vi "Teleop.vi"(10 "Match Info":T1={"Autonomous Elapsed Seconds"=0.0, "TeleOp Elapsed Seconds"=0.0, "Disabled Elapsed Seconds"=0.0, "Visited Autonomous"=FALSE, "Visited TeleOp"=FALSE, "Visited Disabled"=FALSE, "Autonomous Settings"={"Autonomous Style"=enum."Independent", "VI Refnum"=refnum}}, 11 "Call Context":T2) -> ()   [LabVIEW 2014]
doc: "This VI is called for each TeleOp packet received from the DS where the robot is not disabled. It is often used to read from the joysticks and update I/O or to update setpoints for timed control loops. It should complete and return within 20 milliseconds or it may miss DS packets."
uses:
  <vilib>/Rock Robotics/WPI/DriverStation/WPI_DriverStationDerivedRobotMode.ctl
  <vilib>/Rock Robotics/WPI/DriverStation/WPI_DriverStationMatch Info.ctl
  <vilib>/Rock Robotics/Network Tables/SD Read Boolean.vi
  <vilib>/Rock Robotics/Network Tables/SD Read Number.vi
  <vilib>/Rock Robotics/Network Tables/SD Write Numeric Array.vi
panel:
  out "Sample Slider 0":dbl(slide) scale=0.0..5.0
  out "Sample Boolean 1":bool
  out "Sample Boolean 0":bool
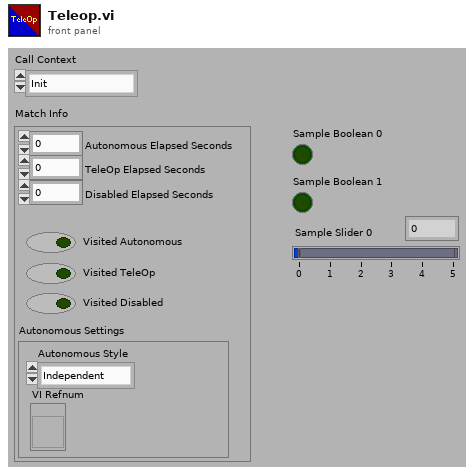
[diagram p1: front panel]
types:
  T1 = typedef "WPI_DriverStationMatch Info.ctl" = cluster{"Autonomous Elapsed Seconds":dbl, "TeleOp Elapsed Seconds":dbl, "Disabled Elapsed Seconds":dbl, "Visited Autonomous":bool, "Visited TeleOp":bool, "Visited Disabled":bool, "Autonomous Settings":cluster{"Autonomous Style":enum16{"Iterative", "Independent"}, "VI Refnum":refnum<vi>}}
  T2 = typedef "WPI_DriverStationDerivedRobotMode.ctl" = enum16{"Init", "Execute", "Stop"}
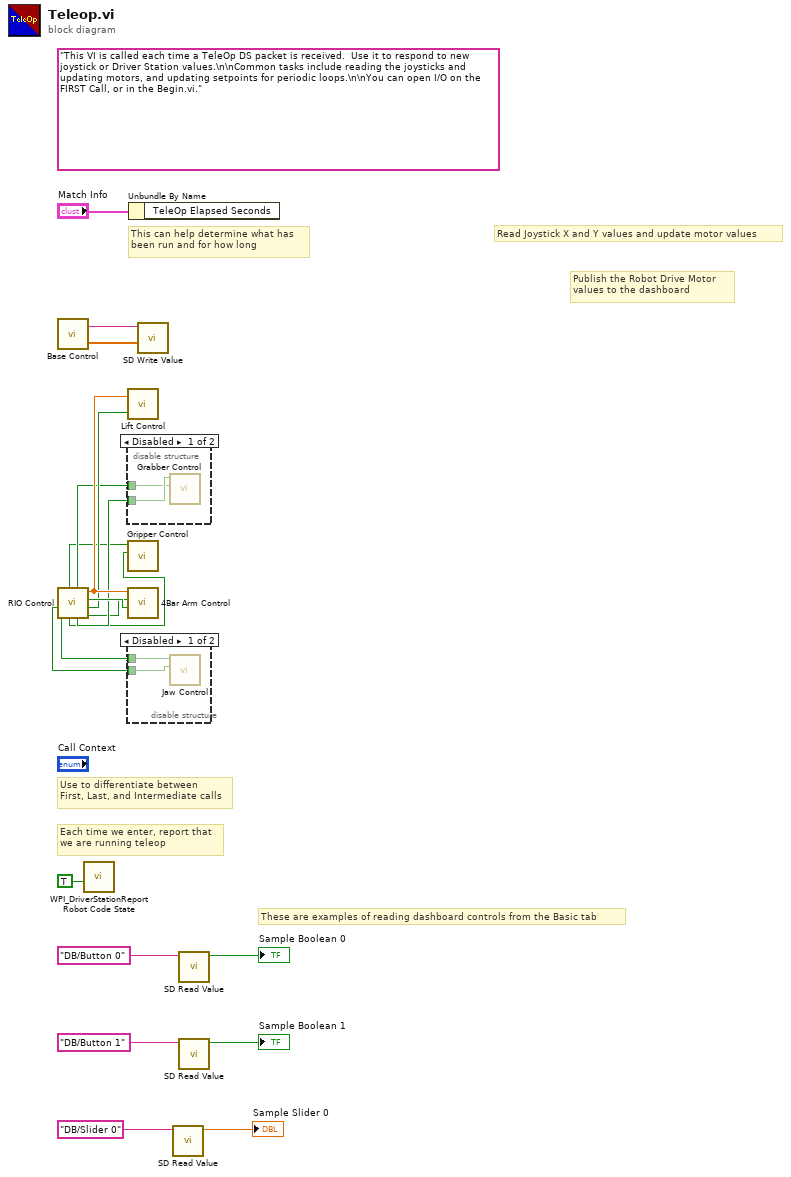
[diagram p0: block diagram]
diagram:
  (unwired) "This VI is called each time a TeleOp DS packet is received.  Use it to respond to new joystick or Driver Station values.\n\nCommon tasks include reading the joysticks and updating motors, and updating setpoints for periodic loops.\n\nYou can open I/O on the FIRST Call, or in the Begin.vi."
  # "These are examples of reading dashboard controls from the Basic tab"
  # "Publish the Robot Drive Motor\nvalues to the dashboard"
  # "Each time we enter, report that\nwe are running teleop"
  # "Use to differentiate between\nFirst, Last, and Intermediate calls"
  # "This can help determine what has\nbeen run and for how long"
  # "Read Joystick X and Y values and update motor values"
  n1 = call "Base Control.vi"() -> ("Name"=w12:string, "Motor Values"=w11:dbl[])  [unwired: 1 in]
  n2 = call "RIO Control.vi"() -> ("Disable Sensors"=w3:bool, "Lift Control"=w8:bool, "4Bar Control"=w10:bool, "Joystick Value"=w9:dbl, "Grabber Inhale"=w7:bool, "Grabber Exhale"=w6:bool, "Close Gripper"=w1:bool, "Open Gripper"=w2:bool, "Jaw Open"=w4:bool, "Jaw Close"=w5:bool)  [unwired: 2 in]
  n3 = call <vilib>:"WPI_DriverStationReport Robot Code State.vi"("TeleOp"=TRUE ("Autonomous")) -> ()  [unwired: 10 in, 1 out]
  n4 = call "Lift Control.vi"("Joystick Input"=w9, "Lift Control"=w8) -> ()  [unwired: 4 in]
  n5 = disable-structure shown="Disabled" {
    disable-tunnel: w7 -> [w22 _]
    disable-tunnel: w6 -> [w21 _]
    frame Disabled {
      n6 = call "Grabber Control.vi"("Arm Motor Exhale Tote"=w21, "Arm Motor Inhale Tote"=w22) -> ()  [unwired: 8 in]
    }
    frame Enabled {
    }
  }
  n7 = call "Gripper Control.vi"("Close Gripper"=w1, "Open Gripper"=w2) -> ()  [unwired: 3 in]
  n8 = call "4Bar Arm Control.vi"("4Bar Button"=w10, "Disable Sensor"=w3, "Joystick Input"=w9) -> ()  [unwired: 9 in]
  n9 = disable-structure shown="Disabled" {
    disable-tunnel: w5 -> [w24 _]
    disable-tunnel: w4 -> [w23 _]
    frame Disabled {
      n10 = call "Jaw Control.vi"("Jaw Close"=w24, "Jaw Open"=w23) -> ()  [unwired: 8 in]
    }
    frame Enabled {
    }
  }
  n11 = Unbundle By Name("Match Info") -> ()  [unwired: 1 out]
  n12 = call-poly <vilib>:"SD Write Value.vi"("Numeric Array"=w11, "Name"=w12) -> ()  [unwired: 8 in, 2 out]
  n13 = call-poly <vilib>:"SD Read Value.vi"("Name"="DB/Slider 0" ("refnum name")) -> ("Numeric"=→"Sample Slider 0":dbl)  [unwired: 8 in, 2 out]
  n14 = call-poly <vilib>:"SD Read Value.vi"("Name"="DB/Button 0" ("refnum name")) -> ("Boolean"=→"Sample Boolean 0":bool)  [unwired: 8 in, 2 out]
  n15 = call-poly <vilib>:"SD Read Value.vi"("Name"="DB/Button 1" ("refnum name")) -> ("Boolean"=→"Sample Boolean 1":bool)  [unwired: 8 in, 2 out]
